vi "Create UID.vi"(0 "Remote Connection Session in":refnum<class "Remote Connection Session.lvclass">, 11 "error in (no error)":errorcluster) -> (4 "Remote Connection Session out":refnum<class "Remote Connection Session.lvclass">, 8 "Session UID":string, 15 "error out":errorcluster)   [LabVIEW 2012, in "REx.lvlib" / "Remote Connection Session.lvclass"]
uses:
  Remote Connection Session.lvclass
  Remote Connection Session.lvclass/Remote Connection Session.ctl
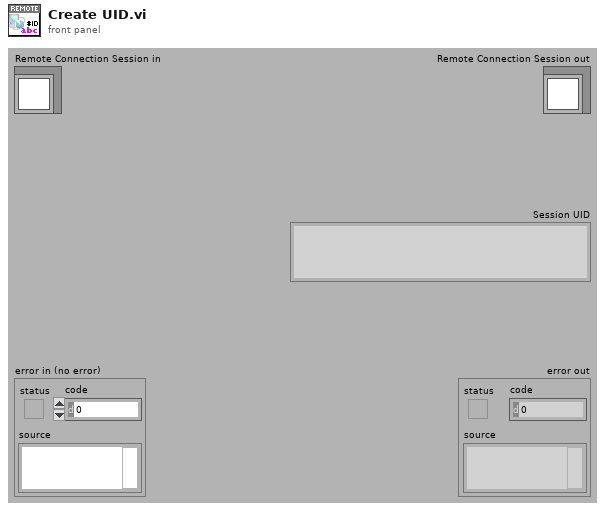
[diagram p1: front panel]
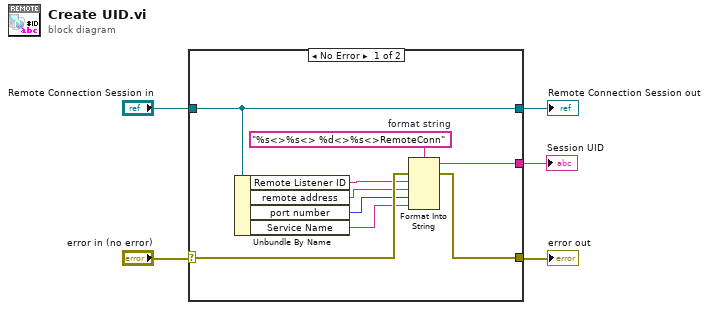
[diagram p0: block diagram]
diagram:
  n1 = case shown="No Error" "error in (no error)" {
    selector: "error in (no error)" -> [w14 w16]
    tunnel: [w7 w16] -> w4
    tunnel: [w13 w15] -> w2
    tunnel: "Remote Connection Session in" -> [w13 w15]
    tunnel: [w9 _] -> w1
    frame No Error {
      w8 = "%s<>%s<> %d<>%s<>RemoteConn"  # format string
      n2 = Unbundle By Name(w13) -> ("Remote Listener ID"=w12:string, "remote address"=w11:string, "port number"=w10:u16, "Service Name"=w6:string)
      n3 = Format Into String(format string=w8, error in=w14, w12, w11, w10, w6) -> (resulting string=w9:string, error out=w7:errorcluster)  [unwired: 1 in]
    }
    frame Error {
    }
  }
  "error out" <- w4
  "Remote Connection Session out" <- w2
  "Session UID" <- w1
